vi "WriteCoreLoop_v2.vi"(5 "InitialFiles Format":T1=enum."Binary Files", 7 "Controls ref.":T2, 8 "data error in":errorcluster, 9 "data queue in":refnum<queue>, 11 "control queue in":refnum<queue>) -> (0 "error out":errorcluster)   [LabVIEW 2014]
uses:
  <instrlib>/GenericDAQ/VI/GenericDAQ_Signal.ctl
  SaveControlsRef.ctl
  WriterState.ctl
  ControlDef/Files_Format.ctl
  <instrlib>/GenericDAQ/GenericDAQ.lvlib
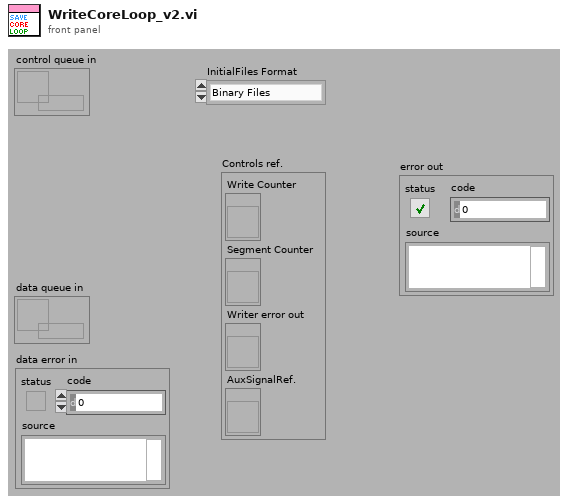
[diagram p1: front panel]
types:
  T1 = typedef "Files_Format.ctl" = enum16{"Text Files", "mzML Files", "Binary Files", "BioMap Files", "imzML Files"}
  T2 = typedef "SaveControlsRef.ctl" = cluster{"Write Counter":refnum<vi>, "Segment Counter":refnum<vi>, "Writer error out":refnum<vi>, "AuxSignalRef.":refnum<vi>}
  T3 = typedef "WriterState.ctl" = cluster{"State":enum16{"Open", "Close", "ChangeFormat", "SetHeader", "QuitProg."}, "Params":variant}
  T4 = enum16{"Open", "Close", "ChangeFormat", "SetHeader", "QuitProg."}
  T5 = typedef "GenericDAQ.lvlib/GenericDAQ_Signal.ctl" = cluster{"tickcount":u32, "Signal":sgl[], "SecondaryData":dbl[], "Flag":enum16{"Normal", "LineStart", "LineEnd", "FrameStart", "FrameEnd", "Reserved1", "Reserved2"}, "Segment#":i32}
  T6 = enum16{"Normal", "LineStart", "LineEnd", "FrameStart", "FrameEnd", "Reserved1", "Reserved2"}
  T7 = typedef "Signal_Segment.ctl" = cluster{"SampleRate":dbl, "TrigDelay":dbl, "SpecLength":dbl, "DAQ_Range":dbl, "Average#":i32, "Position":dbl[], "Spectrum":sgl[], "Calibr.":dbl[], "Pressure":dbl, "Desp_LaserEnergy":dbl, "PI_LaserEnergy":dbl, "Voltages Table":sgl[][], "ProcMode":T8, "Threshold":dbl, "Comment":string, "TickCount":dbl, "Time Stamp":timestamp}
  T8 = typedef "ProcessingMode.ctl" = enum16{"None", "Drop by Threshold", "TDC Simulate", "SetFilter"}
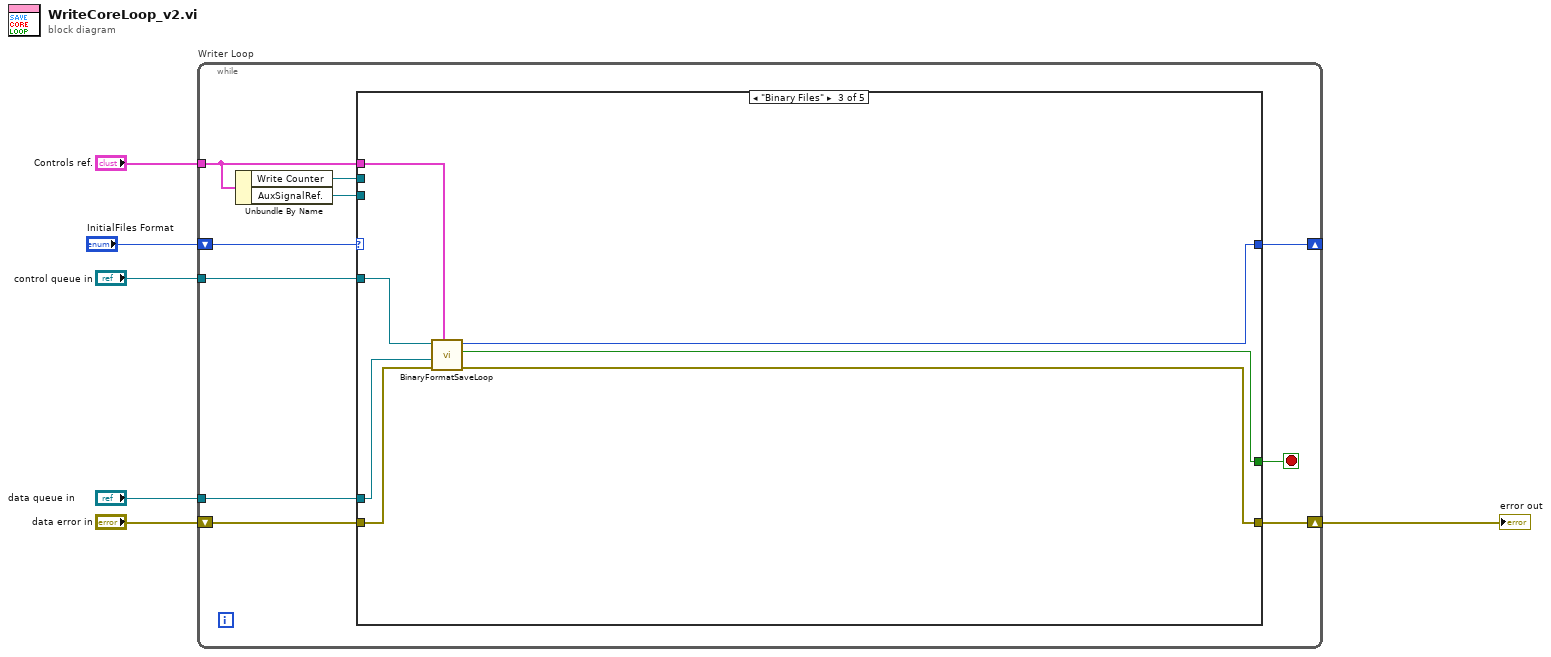
[diagram p0: block diagram]
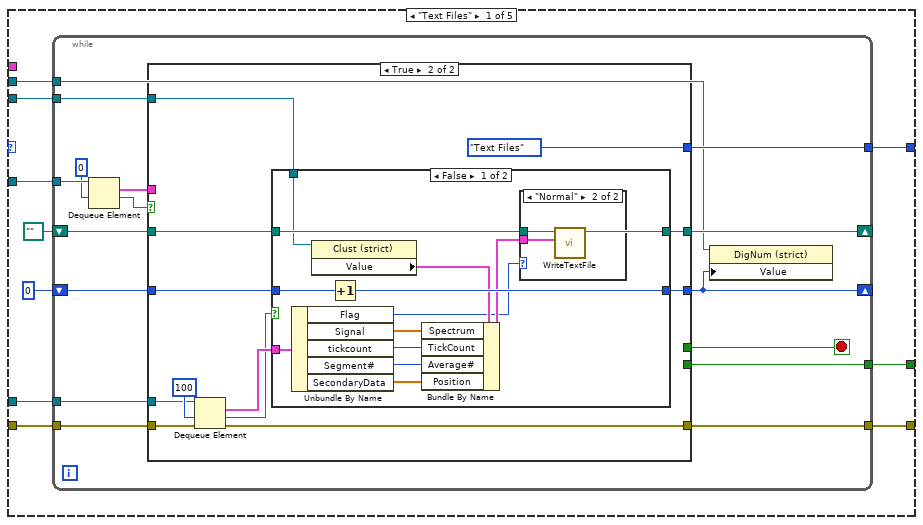
[diagram p2: hidden frame]
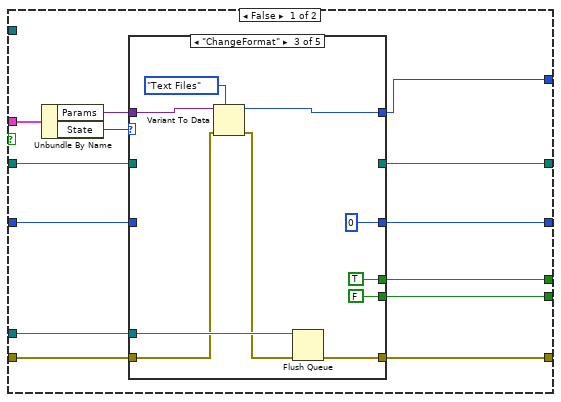
[diagram p3: hidden frame]
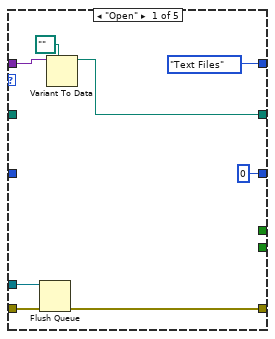
[diagram p4: hidden frame]
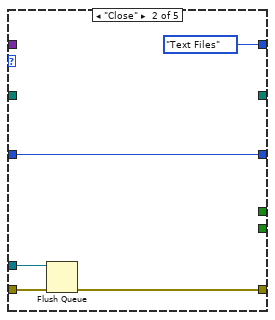
[diagram p5: hidden frame]
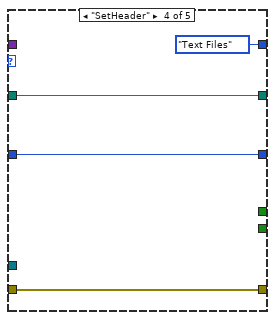
[diagram p6: hidden frame]
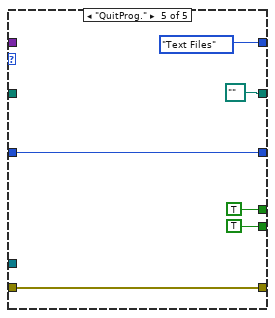
[diagram p7: hidden frame]
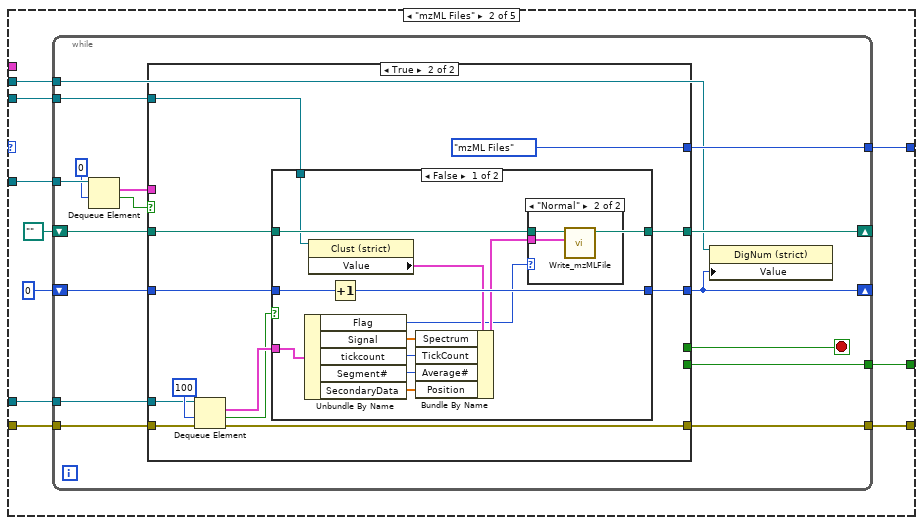
[diagram p10: hidden frame]
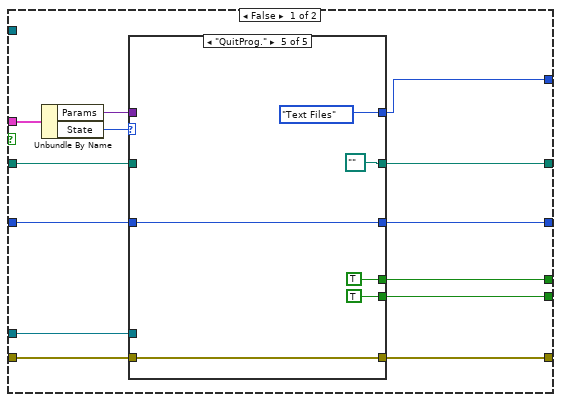
[diagram p11: hidden frame]
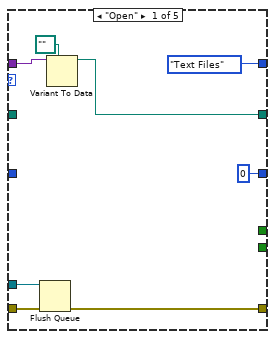
[diagram p12: hidden frame]
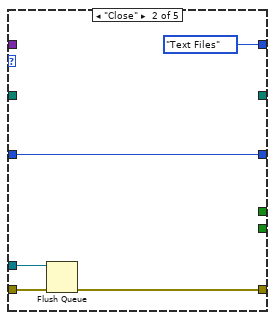
[diagram p13: hidden frame]
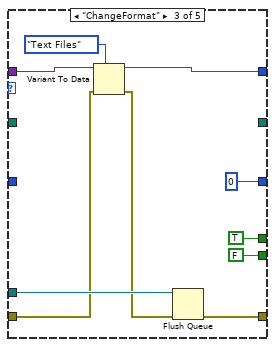
[diagram p14: hidden frame]
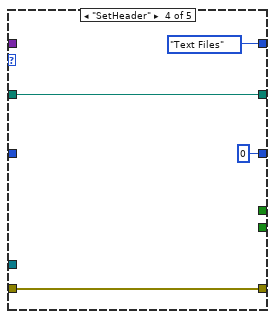
[diagram p15: hidden frame]
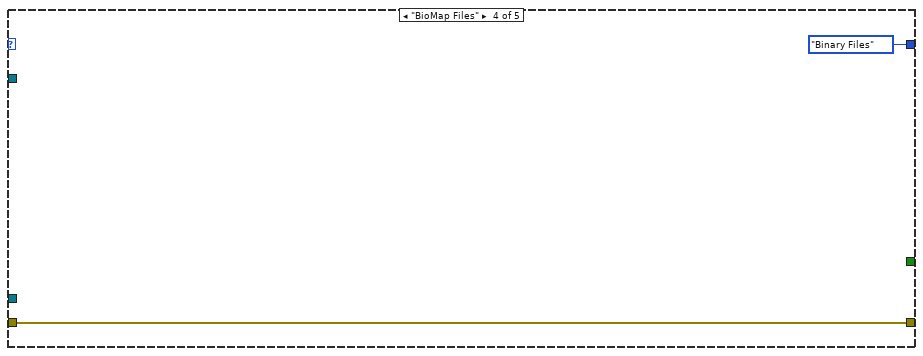
[diagram p18: hidden frame]
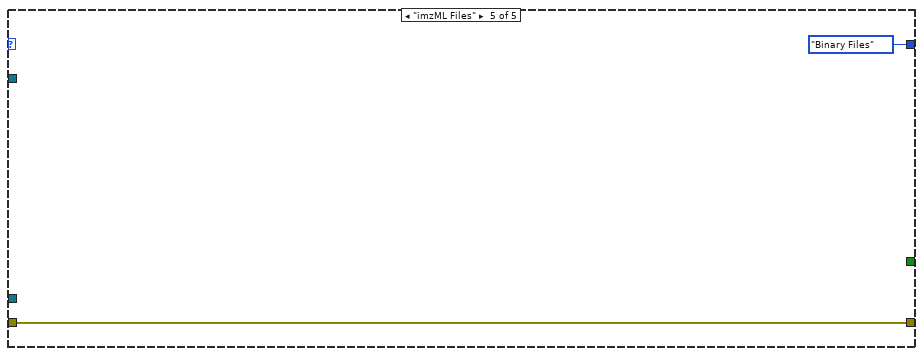
[diagram p19: hidden frame]
diagram:
  n1 = while "Writer Loop" {
    shift-right: [w10] -> w3
    shift-left: "data error in" -> [w14]
    tunnel: "data queue in" -> [w15]
    tunnel: "Controls ref." -> [w9]
    tunnel: "control queue in" -> [w13]
    shift-right: [w11] -> _
    shift-left: "InitialFiles Format" -> [w12]
    stop <- w16 stop-if-true
    n2 = Unbundle By Name(w9) -> ("Write Counter"=w8:refnum<vi>, "AuxSignalRef."=w7:refnum<vi>)
    n3 = case shown="\"Binary Files\"" w12 {
      tunnel: [w26 w126 w223 _ _] -> w16
      tunnel: w15 -> [w24 w124 w222 _ _]
      tunnel: w14 -> [w23 w123 w221 w225 w227]
      tunnel: w13 -> [w22 w122 w220 _ _]
      tunnel: [w21 w121 w219 Files_Format."Binary Files" ("Format") Files_Format."Binary Files" ("Format")] -> w11
      tunnel: [w19 w119 w217 w225 w227] -> w10
      tunnel: w9 -> [_ _ w218 _ _]
      tunnel: w8 -> [w18 w118 _ _ _]
      tunnel: w7 -> [w17 w117 _ _ _]
      frame "Text Files" {
        n4 = while {
          tunnel: [w40] -> w26
          shift-right: [w29] -> _
          shift-left: 0 -> [w42]
          tunnel: w24 -> [w36]
          tunnel: w23 -> [w35]
          shift-right: [w31] -> _
          shift-left: path "" ("file path") -> [w41]
          tunnel: w22 -> [w39]
          tunnel: [w32] -> w21
          tunnel: [w30] -> w19
          tunnel: w18 -> [w28]
          tunnel: w17 -> [w27]
          stop <- w33 stop-if-true
          n5 = Dequeue Element(queue=w39, timeout in ms (-1)=0) -> (element=w34:T3, timed out?=w37:bool)  [unwired: 1 in, 2 out]
          n6 = case shown="True" w37 {
            tunnel: w42 -> [w49 w94]
            tunnel: w41 -> [w53 w96]
            tunnel: [w50 w93] -> w29
            tunnel: [w52 _] -> w40
            tunnel: w36 -> [w47 w99]
            tunnel: w35 -> [w46 w98]
            tunnel: w34 -> [w55 _]
            tunnel: [w51 _] -> w33
            tunnel: [w43 Files_Format."Text Files" ("Format")] -> w32
            tunnel: [w48 w91] -> w31
            tunnel: [w45 w90] -> w30
            tunnel: w27 -> [_ w89]
            frame False {
              n7 = Unbundle By Name(w55) -> ("Params"=w44:variant, "State"=w54:T4)
              n8 = case shown="\"ChangeFormat\"" w54 {
                tunnel: w53 -> [_ _ _ w80 _]
                tunnel: [w56 _ _ w80 path "" ("file path")] -> w48
                tunnel: [_ _ FALSE _ TRUE] -> w52
                tunnel: [_ _ TRUE _ TRUE] -> w51
                tunnel: [Files_Format."Text Files" ("Format") Files_Format."Text Files" ("Format") w72 Files_Format."Text Files" ("Format") Files_Format."Text Files" ("Format")] -> w43
                tunnel: [0 w68 0 w81 w86] -> w50
                tunnel: w49 -> [_ w68 _ w81 w86]
                tunnel: w47 -> [w60 w66 w75 _ _]
                tunnel: w46 -> [w61 w67 w70 w79 w83]
                tunnel: [w59 w65 w74 w79 w83] -> w45
                tunnel: w44 -> [w57 _ w73 _ _]
                frame "Open" {
                  n9 = Flush Queue(queue=w60, error in (no error)=w61) -> (error out=w59:errorcluster)  [unwired: 2 out]
                  n10 = Variant To Data(type=path "" ("path"), Variant=w57) -> (data=w56:path)  [unwired: 1 in, 1 out]
                }
                frame "Close" {
                  n11 = Flush Queue(queue=w66, error in (no error)=w67) -> (error out=w65:errorcluster)  [unwired: 2 out]
                }
                frame "ChangeFormat" {
                  n12 = Variant To Data(error in=w70, type=Files_Format."Text Files" ("Format"), Variant=w73) -> (data=w72:T1, error out=w71:errorcluster)
                  n13 = Flush Queue(queue=w75, error in (no error)=w71) -> (error out=w74:errorcluster)  [unwired: 2 out]
                }
                frame "SetHeader" {
                }
                frame "QuitProg." {
                }
              }
            }
            frame True {
              n14 = Dequeue Element(queue=w99, timeout in ms (-1)=100, error in (no error)=w98) -> (element=w97:T5, timed out?=w92:bool, error out=w90:errorcluster)  [unwired: 1 out]
              n15 = case shown="False" w92 {
                tunnel: w97 -> [w105 _]
                tunnel: w96 -> [w112 w116]
                tunnel: [w112 w116] -> w91
                tunnel: w94 -> [w111 w115]
                tunnel: [w110 w115] -> w93
                tunnel: w89 -> [w103 _]
                frame False {
                  n16 = Unbundle By Name(w105) -> ("Flag"=w101:T6, "Signal"=w109:sgl[], "tickcount"=w108:u32, "Segment#"=w102:i32, "SecondaryData"=w107:dbl[])
                  n17 = property class="Clust (strict)"(reference=w103) -> ("Value"=w104:T7)  [unwired: 1 in, 2 out]
                  n18 = Increment(x=w111) -> (x+1=w110:i32)
                  n19 = Bundle By Name(cluster=w104, "Spectrum"=w109, "TickCount"=w108, "Average#"=w102, "Position"=w107) -> (w106:T7)
                  n20 = case shown="\"Normal\"" w101 {
                    tunnel: w112 -> [_ w114]
                    tunnel: w106 -> [_ w113]
                    frame Default {
                    }
                    frame "Normal" {
                      n21 = call "WriteTextFile.vi"("Signal Segment"=w113, "Filename"=w114) -> ()  [unwired: 9 in, 1 out]
                    }
                  }
                }
                frame True {
                }
              }
            }
          }
          n22 = property class="DigNum (strict)"(reference=w28, "Value"=w29) -> ()  [unwired: 1 in, 2 out]
        }
      }
      frame "mzML Files" {
        n23 = while {
          tunnel: [w140] -> w126
          shift-right: [w129] -> _
          shift-left: 0 -> [w142]
          tunnel: w124 -> [w136]
          tunnel: w123 -> [w135]
          shift-right: [w131] -> _
          shift-left: path "" ("file path") -> [w141]
          tunnel: w122 -> [w139]
          tunnel: [w132] -> w121
          tunnel: [w130] -> w119
          tunnel: w118 -> [w128]
          tunnel: w117 -> [w127]
          stop <- w133 stop-if-true
          n24 = Dequeue Element(queue=w139, timeout in ms (-1)=0) -> (element=w134:T3, timed out?=w137:bool)  [unwired: 1 in, 2 out]
          n25 = case shown="True" w137 {
            tunnel: w142 -> [w149 w194]
            tunnel: w141 -> [w153 w196]
            tunnel: [w150 w193] -> w129
            tunnel: [w152 _] -> w140
            tunnel: w136 -> [w147 w199]
            tunnel: w135 -> [w146 w198]
            tunnel: w134 -> [w155 _]
            tunnel: [w151 _] -> w133
            tunnel: [w143 Files_Format."mzML Files" ("Format")] -> w132
            tunnel: [w148 w191] -> w131
            tunnel: [w145 w190] -> w130
            tunnel: w127 -> [_ w189]
            frame False {
              n26 = Unbundle By Name(w155) -> ("Params"=w144:variant, "State"=w154:T4)
              n27 = case shown="\"QuitProg.\"" w154 {
                tunnel: w153 -> [_ _ _ w180 _]
                tunnel: [w156 _ _ w180 path "" ("file path")] -> w148
                tunnel: [_ _ FALSE _ TRUE] -> w152
                tunnel: [_ _ TRUE _ TRUE] -> w151
                tunnel: [Files_Format."Text Files" ("Format") Files_Format."Text Files" ("Format") w172 Files_Format."Text Files" ("Format") Files_Format."Text Files" ("Format")] -> w143
                tunnel: [0 w168 0 0 w186] -> w150
                tunnel: w149 -> [_ w168 _ _ w186]
                tunnel: w147 -> [w160 w166 w175 _ _]
                tunnel: w146 -> [w161 w167 w170 w179 w185]
                tunnel: [w159 w165 w174 w179 w185] -> w145
                tunnel: w144 -> [w157 _ w173 _ _]
                frame "Open" {
                  n28 = Flush Queue(queue=w160, error in (no error)=w161) -> (error out=w159:errorcluster)  [unwired: 2 out]
                  n29 = Variant To Data(type=path "" ("path"), Variant=w157) -> (data=w156:path)  [unwired: 1 in, 1 out]
                }
                frame "Close" {
                  n30 = Flush Queue(queue=w166, error in (no error)=w167) -> (error out=w165:errorcluster)  [unwired: 2 out]
                }
                frame "ChangeFormat" {
                  n31 = Variant To Data(error in=w170, type=Files_Format."Text Files" ("Format"), Variant=w173) -> (data=w172:T1, error out=w171:errorcluster)
                  n32 = Flush Queue(queue=w175, error in (no error)=w171) -> (error out=w174:errorcluster)  [unwired: 2 out]
                }
                frame "SetHeader" {
                }
                frame "QuitProg." {
                }
              }
            }
            frame True {
              n33 = Dequeue Element(queue=w199, timeout in ms (-1)=100, error in (no error)=w198) -> (element=w197:T5, timed out?=w192:bool, error out=w190:errorcluster)  [unwired: 1 out]
              n34 = case shown="False" w192 {
                tunnel: w197 -> [w208 _]
                tunnel: w196 -> [w212 w216]
                tunnel: [w212 w216] -> w191
                tunnel: w194 -> [w211 w215]
                tunnel: [w210 w215] -> w193
                tunnel: w189 -> [w202 _]
                frame False {
                  n35 = Unbundle By Name(w208) -> ("Flag"=w201:T6, "Signal"=w207:sgl[], "tickcount"=w206:u32, "Segment#"=w205:i32, "SecondaryData"=w204:dbl[])
                  n36 = property class="Clust (strict)"(reference=w202) -> ("Value"=w203:T7)  [unwired: 1 in, 2 out]
                  n37 = Increment(x=w211) -> (x+1=w210:i32)
                  n38 = Bundle By Name(cluster=w203, "Spectrum"=w207, "TickCount"=w206, "Average#"=w205, "Position"=w204) -> (w209:T7)
                  n39 = case shown="\"Normal\"" w201 {
                    tunnel: w212 -> [_ w214]
                    tunnel: w209 -> [_ w213]
                    frame Default {
                    }
                    frame "Normal" {
                      n40 = call "Write_mzMLFile.vi"("Signal Segment"=w213, "Filename"=w214) -> ()  [unwired: 9 in, 1 out]
                    }
                  }
                }
                frame True {
                }
              }
            }
          }
          n41 = property class="DigNum (strict)"(reference=w128, "Value"=w129) -> ()  [unwired: 1 in, 2 out]
        }
      }
      frame "Binary Files" {
        n42 = call "BinaryFormatSaveLoop.vi"("Controls ref."=w218, "data error in"=w221, "data queue in"=w222, "control queue in"=w220) -> ("queue error out"=w217:errorcluster, "Quit Binary"=w223:bool, "Format"=w219:T1)  [unwired: 4 in, 1 out]
      }
      frame "BioMap Files" {
      }
      frame "imzML Files" {
      }
    }
  }
  "error out" <- w3
